vi "UsrProfiles-Remove user key.vi"(8 "error in (no error)":errorcluster, 11 "Name of user to remove":string) -> ()   [LabVIEW 2013]
uses:
  Typedefs/Which path.ctl
  <vilib>/Utility/config.llb/NI_LVConfig.lvlib
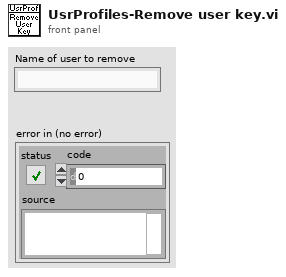
[diagram p1: front panel]
types:
  T1 = typedef "Which path.ctl" = enum16{"Configuration Files", "Calibration Files", "Images", "Setup.ini", "Loaded User profile.ini", "User's-Previous session.ini", "New user profile.ini", "Selected User profile.ini", "User profiles folder", "Power meter scaling.txt", "FOV Cal.ini"}
  T2 = typedef "NI_LVConfig.lvlib/Config Data RefNum.ctl" = refnum<k1>
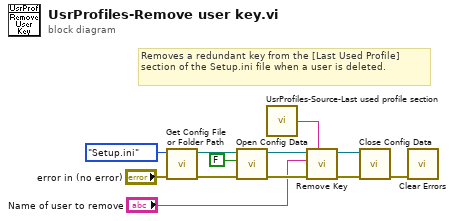
[diagram p0: block diagram]
diagram:
  # "Removes a redundant key from the [Last Used Profile] section of the Setup.ini file when a user is deleted."
  n1 = call "Get Config File or Folder Path.vi"("Error In"="error in (no error)", "Which file or folder?"=Which_path."Setup.ini") -> ("Error Out"=w8:errorcluster, "File Path"=w10:path)  [unwired: 7 in, 1 out]
  n2 = call <vilib>:"Open Config Data.vi"("error in (no error)"=w8, "create file if necessary (T)"=FALSE, "configuration file path"=w10) -> ("error out"=w6:errorcluster, "refnum"=w7:T2)  [unwired: 6 in, 1 out]
  n3 = call "UsrProfiles-Source-Last used profile section.vi"() -> ("Last Used Profile section name"=w1:string)  [unwired: 1 in]
  n4 = call <vilib>:"Remove Key.vi"("section"=w1, "error in (no error)"=w6, "key"="Name of user to remove", "refnum"=w7) -> ("error out"=w4:errorcluster, "refnum out"=w3:T2)  [unwired: 5 in, 1 out]
  n5 = call <vilib>:"Close Config Data.vi"("error in (no error)"=w4, "refnum"=w3) -> ("error out"=w2:errorcluster)  [unwired: 8 in, 1 out]
  n6 = call <vilib>:"Clear Errors.vi"("error in (no error)"=w2) -> ()  [unwired: 6 in, 1 out]
